vi "Read Position.vi"(8 "error in (no error)":errorcluster, 11 "Transform in":refnum<class "Transform.lvclass">) -> (0 "error out":errorcluster, 2 "Position out":refnum<class "Vector2.lvclass">, 3 "Transform out":refnum<class "Transform.lvclass">)   [LabVIEW 2022 SP3, in "Transform.lvclass"]
uses:
  Transform.lvclass
  Math/Vector2/Vector2.lvclass
  Transform.lvclass/Transform.ctl
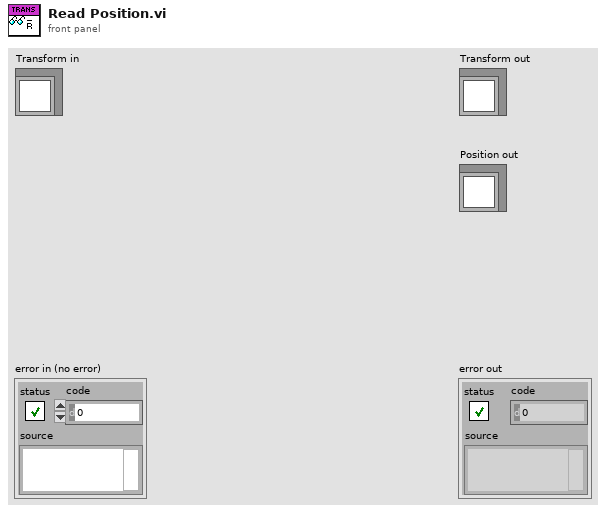
[diagram p1: front panel]
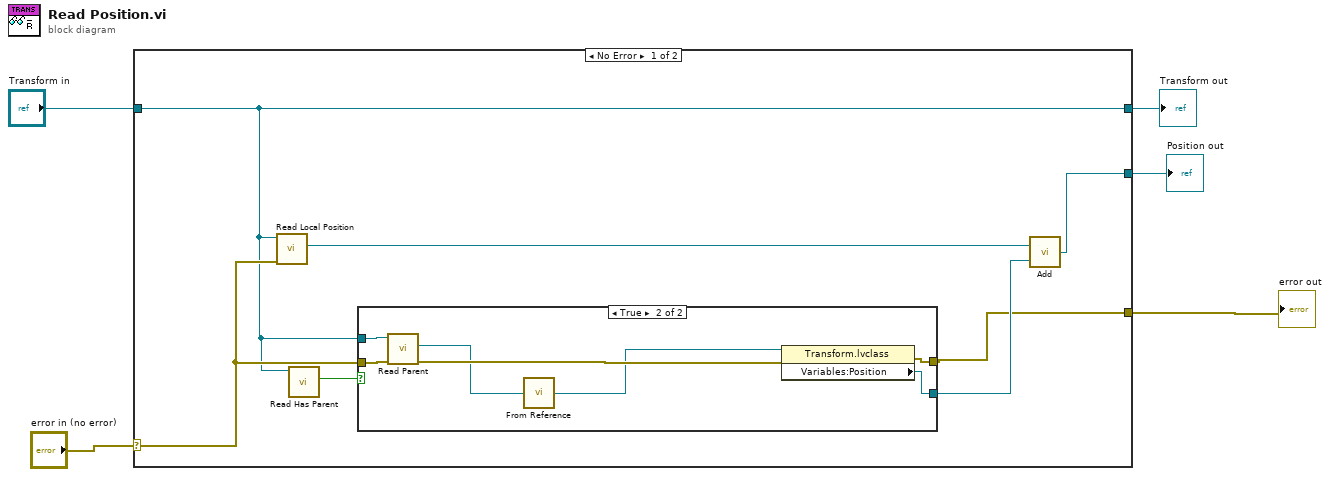
[diagram p0: block diagram]
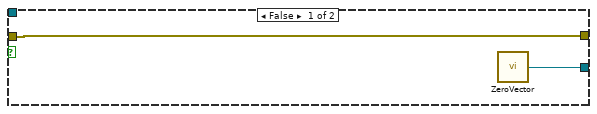
[diagram p2: hidden frame]
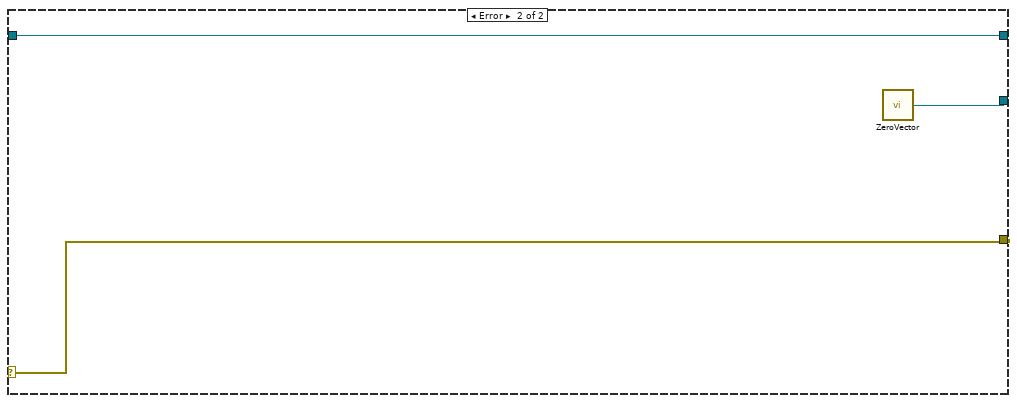
[diagram p3: hidden frame]
diagram:
  n1 = case shown="No Error" "error in (no error)" {
    selector: "error in (no error)" -> [w12 w22]
    tunnel: [w7 w24] -> w3
    tunnel: "Transform in" -> [w7 w24]
    tunnel: [w9 w23] -> w2
    tunnel: [w6 w22] -> w1
    frame No Error {
      n2 = call "Read Local Position.vi"("error in (no error)"=w12, "Transform in"=w7) -> ("Local Position out"=w11:refnum<class "Vector2.lvclass">)  [unwired: 7 in, 2 out]
      n3 = call "Read Has Parent.vi"("Transform in"=w7) -> ("Has Parent"=w8:bool)  [unwired: 8 in, 2 out]
      n4 = case shown="True" w8 {
        tunnel: w12 -> [w13 w21]
        tunnel: w7 -> [_ w20]
        tunnel: [w14 w19] -> w10
        tunnel: [w13 w18] -> w6
        frame False {
          n5 = call "ZeroVector.vi"() -> ("Zero Vector"=w14:refnum<class "Vector2.lvclass">)
        }
        frame True {
          n6 = call "Read Parent.vi"("error in (no error)"=w21, "Transform in"=w20) -> ("error out"=w17:errorcluster, "Parent"=w16:refnum<vi>)  [unwired: 7 in, 1 out]
          n7 = call "From Reference.vi"("Transform Ref in"=w16) -> ("Transform out"=w15:refnum<class "Transform.lvclass">)
          n8 = property class="Transform.lvclass"(reference=w15, error in=w17) -> (error out=w18:errorcluster, "Variables:Position"=w19:refnum<class "Vector2.lvclass">)  [unwired: 1 out]
        }
      }
      n9 = call "Add.vi"("Vec2 b in"=w10, "Vec2 a in"=w11) -> ("Vec2 out"=w9:refnum<class "Vector2.lvclass">)
    }
    frame Error {
      n10 = call "ZeroVector.vi"() -> ("Zero Vector"=w23:refnum<class "Vector2.lvclass">)
    }
  }
  "error out" <- w1
  "Transform out" <- w3
  "Position out" <- w2
